vi "AlliGator Global Decay Fit Output String.vi"(0 "Plot Names":string[](array[string]), 5 "Fit Output":T2={"best nonlinear fit"=[], "best fit parameters"=[], "R^2"=0.0, "RMSE"=0.0, "error out"={"status"=FALSE, "code"=0, "source"=""}, "Fitting Method"=enum."Least Square", "number of function calls"=0, "number of iterations"=0, "covariance"=[], "Chi 2"=0.0, "DOF"=0, "Fit Convergence Criterion"=enum."Continue", "Fitting Algorithm"=enum."Levenberg-Marquardt", "Weighted Fit"=enum."Unweighted", "Gradient"=0.0, "|Delta Chi 2|"=0.0, "|Delta Chi 2|/Chi 2"=0.0, "Max |Delta a| /|a|"=0.0, "Lambda"=-1.0, "RSS"=0.0, "AIC"=0.0, "BIC"=0.0, "Max number of function calls"=0, "Max number of iterations"=0, "IRF"={"X Array"=[], "Y Array"=[]}, "IRF Normalization Factor"=0.0, "Decay Normalization Factor"=0.0, "Number of offset fits"=0, "Weighted Chi2"=-1.0, "Unweighted Chi2"=-1.0}, 7 "Delta Best Fit Parameters":dbl[](array[numeric]), 9 "elapsed (relative) seconds":dbl, 11 "Error In":errorcluster, 12 "Fit Options":T9={"Show Fit Residuals"=TRUE, "Fit Model"=enum."1-Exponential", "Residual Type"=enum."Standard", "Max Decay Percentile"=0.0, "Min Decay Percentile"=0.0, "Show Full Decay"=TRUE, "Weights"=enum."Unweighted", "Fitting Method"=enum."Least Square", "Compute Parameter Uncertainties"=TRUE, "Periodic Boundaries"=TRUE, "Model Calculation"=enum."Simulation", "Period"=1.2500000000000001e-08, "Termination Criteria"={"Max Iterations"=1000, "Max Function Calls"=0, "Max Time"=1000.0, "Function Tolerance"=1e-06, "Parameter Tolerance"=1e-06, "Gradient Tolerance"=0.0, "Min Lambda"=1e-06, "Max Lambda"=1e-06, "Initial Tick Count"=0}, "Offset Resolution"=1.2500000000000001e-08, "Use Local IRF"=TRUE, "Fitting Algorithm"=enum."Levenberg-Marquardt", "Show Confidence Interval "=TRUE, "Confidence Level"=95.0} {"Confidence Level" min=0.0 max=100.0; "Offset Resolution" min=0.0; "Period" min=0.0; "Min Decay Percentile" min=0.0 max=1.0; "Max Decay Percentile" min=0.0 max=100.0}, 13 "Fit Parameter Constraints":T14[](array[typedef]) {"Max Value" format="%#.3g"; "Min Value" format="%#.3g"}, 14 "Global Fit Parameter Info":T8) -> (4 "Fit Output Message":string, 15 "Error Out":errorcluster)   [LabVIEW 2021, in "AlliGator Global Decay Fit.lvlib"]
uses:
  AlliGator Global Decay Fit.lvlib
  Decay Fit/AlliGator Decay Fit Parameter Constraints 2.ctl
  Fits/IRF(X)PSED/Decay Fit Parameters In List.ctl
  Fits/Decay Convolution/Decay Model.ctl
  Fits/Residual Type.ctl
  Fits/Non-linear Fitting Method v2.ctl
  Fits/Fit Calculation Method.ctl
  Fits/Non-linear Fitting Algorithm.ctl
  Fits/Global Fits/Global Fit Parameters Information.ctl
  Fits/Non-linear Fit Output v4.ctl
  Fits/Nonlinear Fit Method.ctl
  <vilib>/Analysis/Matrix/Datatypes/RealMatrix.ctl
  Fits/Convergence Criteria.ctl
  Fits/IRF(X)PSED/Fit Weights Type v2.ctl
  Graphs/XY Graph/XY Graph Plot Data.ctl
  Settings/AlliGator Settings List.ctl
  <vilib>/Utility/error.llb/DialogType.ctl
  dade2e8c-81fa-42a5-b12d-40fd9ae52111.vi
  Variant/Variant to Data/Variant to Boolean.vi
  <vilib>/Utility/libraryn.llb/Get File Extension.vi
  <vilib>/Utility/error.llb/Error Cluster From Error Code.vi
  <vilib>/ErrorRing/Error Ring.xnode
  Fits/Fits.lvlib
  Strings/Strings.lvlib
  Settings/AlliGator Settings.lvlib
  Variant/Variant to Data/Variant to Data.lvlib
  Sound/Sound.lvlib
  Decay Fit/AlliGator Decay Fit.lvlib
  <vilib>/Analysis/Matrix/NI_Matrix.lvlib
  Graphs/XY Graph/XY Graph Add-Ons.lvlib
  Fits/IRF(X)PSED/Decay Fit Options v4.ctl
panel:
  in  "NL Fit Method":T1
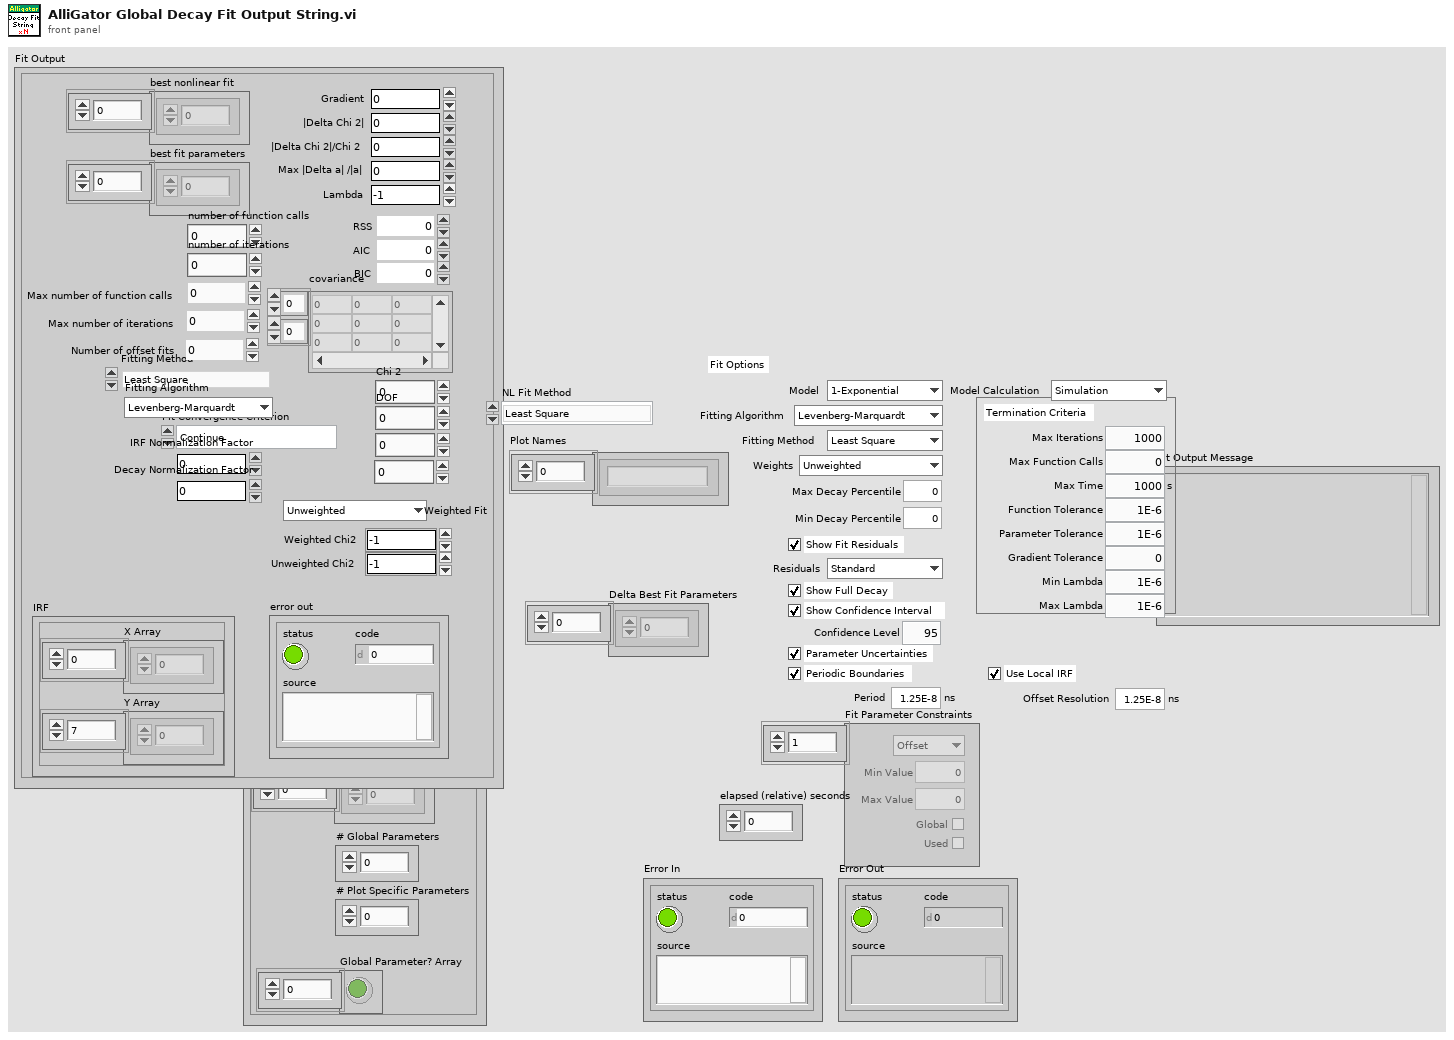
[diagram p1: front panel]
types:
  T1 = typedef "Fits.lvlib/Nonlinear Fit Method.ctl" = enum16{"Least Square", "Least Absolute Residual", "Bisquare", "MLE"}
  T2 = typedef "Fits.lvlib/Non-linear Fit Output v4.ctl" = cluster{"best nonlinear fit":dbl[], "best fit parameters":dbl[], "R^2":dbl, "RMSE":dbl, "error out":errorcluster, "Fitting Method":T1, "number of function calls":i32, "number of iterations":i32, "covariance":T3, "Chi 2":dbl, "DOF":i32, "Fit Convergence Criterion":T4, "Fitting Algorithm":T5, "Weighted Fit":T6, "Gradient":dbl, "|Delta Chi 2|":dbl, "|Delta Chi 2|/Chi 2":dbl, "Max |Delta a| /|a|":dbl, "Lambda":dbl, "RSS":dbl, "AIC":dbl, "BIC":dbl, "Max number of function calls":i32, "Max number of iterations":i32, "IRF":T7, "IRF Normalization Factor":dbl, "Decay Normalization Factor":dbl, "Number of offset fits":i32, "Weighted Chi2":dbl, "Unweighted Chi2":dbl}
  T3 = typedef "NI_Matrix.lvlib/RealMatrix.ctl" = dbl[][]
  T4 = typedef "Fits.lvlib/Convergence Criteria.ctl" = enum16{"Continue", "Tolerances Exceeded", "Max Time Exceeded", "Max Iterations Exceeded", "Max Function Evaluations Exceeded", "Scale Range Exceeded"}
  T5 = typedef "Fits.lvlib/Non-linear Fitting Algorithm.ctl" = enum16{"Levenberg-Marquardt", "Trust-Region Dogleg"}
  T6 = typedef "Fits.lvlib/Fit Weights Type v2.ctl" = enum16{"Unweighted", "1/Variance (Neyman)", "1/Variance (Pearson)", "Best of All"}
  T7 = typedef "XY Graph Add-Ons.lvlib/XY Graph Plot Data.ctl" = cluster{"X Array":dbl[], "Y Array":dbl[]}
  T8 = typedef "Fits.lvlib/Global Fit Parameters Information.ctl" = cluster{"Original Parameter Indices":i32[], "# Global Parameters":i32, "# Plot Specific Parameters":i32, "Global Parameter? Array":bool[]}
  T9 = typedef "Fits.lvlib/Decay Fit Options v4.ctl" = cluster{"Show Fit Residuals":bool, "Fit Model":T10, "Residual Type":T11, "Max Decay Percentile":dbl, "Min Decay Percentile":dbl, "Show Full Decay":bool, "Weights":T6, "Fitting Method":T12, "Compute Parameter Uncertainties":bool, "Periodic Boundaries":bool, "Model Calculation":T13, "Period":dbl[unit], "Termination Criteria":cluster{"Max Iterations":i32, "Max Function Calls":i32, "Max Time":dbl[unit], "Function Tolerance":dbl, "Parameter Tolerance":dbl, "Gradient Tolerance":dbl, "Min Lambda":dbl, "Max Lambda":dbl, "Initial Tick Count":u32}, "Offset Resolution":dbl[unit], "Use Local IRF":bool, "Fitting Algorithm":T5, "Show Confidence Interval ":bool, "Confidence Level":dbl}
  T10 = typedef "Fits.lvlib/Decay Model.ctl" = enum16{"1-Exponential", "2-Exponentials"}
  T11 = typedef "Fits.lvlib/Residual Type.ctl" = enum16{"Standard", "Normalized", "Reduced"}
  T12 = typedef "Fits.lvlib/Non-linear Fitting Method v2.ctl" = enum16{"Least Square", "Least Absolute Residual", "Bisquare", "MLE", "-", "Best of All"}
  T13 = typedef "Fits.lvlib/Fit Calculation Method.ctl" = enum16{"Simulation", "Convolution", "Integration"}
  T14 = typedef "AlliGator Decay Fit.lvlib/AlliGator Decay Fit Parameter Constraints 2.ctl" = cluster{"Fit Parameter":T15, "Min Value":dbl, "Max Value":dbl, "Global":bool, "Used":bool}
  T15 = typedef "Fits.lvlib/Decay Fit Parameters In List.ctl" = enum16{"Offset", "Baseline", "A_1", "tau_1", "A_2", "tau_2"}
  T16 = typedef "AlliGator Settings.lvlib/AlliGator Settings List.ctl" = enum16{"GUI:Visible Settings Tab", "GUI:Last Run Version", "Source Image:Use Image Histogram for Contrast", "Source Image:Low Count Pixels Rejection Options", "Source Image:High Count Pixels Rejection Options", "Source Image:Use Image Brightness", "Source Image:Blend Overlay with Image Background", "Source Image:Use Fixed ROI Diameter", "Source Image:ROI Diameter", "Source Image:ROI Center Color", "Source Image:Peak Threshold", "Source Image:Intensity Threshold", "Source Image:Image Binning Options", "Source Image:Image Smoothing Options", "Source Image:Image Histogram Active", "Source Image:Invert Binary Mask", "Source Image:Hot Pixel Removal", "Source Image:Overlay Analyzed ROI Center", "Source Image:Auto-Adjust Contrast", "Source Image:Histogram Lower Percentile", "Source Image:Histogram Upper Percentile", "Source Image:Save Source Image", "Source Image:Scale Bar Options", "Source Image:Image Resolution (Pixel Size)", "Source Image:Flatfield Correction", "Source Image:Show Dead Left Columns Correction", "Source Image:Dead Left Columns Correction", "Source Image:Image Pre-Processing Operations Order", "Source Image:Overlay ROI Median", "Source Image:Median Overlay Color", "Data Information:Gate Width", "Data Information:Nanotime Gate Separation", "Data Information:Macrotime Gate Separation", "Data Information:Gate Step", "Data Information:# Gates", "Data Information:Gate Image Exposure", "Data Information:Gate Image Integration", "Data Information:Gates to Skip", "Data Information:Gates to Keep", "Data Information:Define Gates to", "Data Information:Channel Name", "Data Information:Available Channel Names", "Data Information:Channel Arithmetic", "Data Information:Background File Subtraction", "Data Information:Background File", "Data Information:Background Scaling Factor", "Data Information:Background Pile-up Correction", "Data Information:Background Pixel Well Capacity", "Data Information:Laser Period", "Data Information:SYNC Period", "Data Information:Pile-up Correction", "Data Information:Pixel Well Capacity", "Data Information:Dataset Scaling Factor", "Fluorescence Decay_Decay Pre-Processing:Reverse Gates", "Fluorescence Decay_Decay Pre-Processing:Verbose Decay Pre-Processing", "Fluorescence Decay_Decay Pre-Processing:Use Decay Pre-Processing", "Fluorescence Decay_Decay Pre-Processing:Background Subtraction", "Fluorescence Decay_Decay Pre-Processing:Background Definition Range", "Fluorescence Decay_Decay Pre-Processing:Baseline Subtraction Method", "Fluorescence Decay_Decay Pre-Processing:Decay Pre-Processing Operations Order", "Fluorescence Decay_Decay Pre-Processing:Smoothing Parameter", "Fluorescence Decay_Decay Pre-Processing:Shift Decay", "Fluorescence Decay_Decay Pre-Processing:Decay Shift Parameters", "Fluorescence Decay_Decay Pre-Processing:Fold Decay", "Fluorescence Decay_Decay Pre-Processing:# Folds", "Fluorescence Decay_Decay Pre-Processing:1-Normalize Decay", "Fluorescence Decay_Decay Pre-Processing:[0-1]-Normalize Decay", "Fluorescence Decay_Decay Pre-Processing:Smoothen Decay", "Fluorescence Decay_Decay Pre-Processing:Extrapolate Decay", "Fluorescence Decay_Decay Pre-Processing:Use Periodicity", "Fluorescence Decay_Decay Pre-Processing:Use Cursors", "Fluorescence Decay_Decay Pre-Processing:Tail Fraction", "Fluorescence Decay_Decay Pre-Processing:Head Fraction", "Fluorescence Decay_Decay Pre-Processing:Additional Points", "Fluorescence Decay_Decay Pre-Processing:Straighten Decay", "Fluorescence Decay_Decay Pre-Processing:Constant Background", "Fluorescence Decay_Decay Pre-Processing:Pixel-Normalize Decay", "Fluorescence Decay_Advanced Analysis:Extract IRF instead of Decay", "Fluorescence Decay_Advanced Analysis:IRF Extraction Options", "Fluorescence Decay_Advanced Analysis:IRF Optimization Options", "Fluorescence Decay_Advanced Analysis:Square Pulse Options", "Fluorescence Decay_Advanced Analysis:IRF Order", "Fluorescence Decay_Advanced Analysis:IRF Time Constants", "Fluorescence Decay_Advanced Analysis:Wavelet Analysis Options", "Fluorescence Decay_Advanced Analysis:Average Lifetime Options", "Fluorescence Decay_Fit Options:Fit Options", "Fluorescence Decay_Fit Options:Use Legacy Fitting Approach", "Fluorescence Decay_Fit Options:Use Data Information Laser Period", "Fluorescence Decay_Fit Parameters:Displayed Fit Parameters", "Fluorescence Decay_Fit Parameters:Fit Parameter Constraints", "Fluorescence Decay_Fit Parameters:Export Tabulated Results", "Fluorescence Decay_Fit Parameters:MLE Baseline Offset Type", "Fluorescence Decay_Fit Parameters:MLE Baseline Offset", "Fluorescence Decay_Fit Parameters:Guess Parameter Names", "Fluorescence Decay_Fit Parameters:Guess Parameter Values", "Fluorescence Decay_Fit Parameters:Guess Parameters Options", "Fluorescence Decay_Fit Parameters:Optimal Offset Selection Criterion", "Fluorescence Decay_Styles:Show Last Decay Only", "Fluorescence Decay_Styles:Decay Graph Color Array", "Fluorescence Decay:Decay Graph Active", "Fluorescence Decay Statistics:Min Peak Value", "Fluorescence Decay Statistics:Reject Low Decay Peak Pixels", "Fluorescence Decay Statistics:Reject High Decay Peak Pixels", "Fluorescence Decay Statistics:Max Peak Value", "Time Traces:Use File Timestamp", "Time Traces:Time Step", "Time Traces:Use Intensity Correction File", "Time Traces:Intensity Correction File", "Phasor Plot:Phasor Plot Smoothing Options", "Phasor Plot:Phasor Plot Size", "Phasor Plot:Phasor Plot Graphics Options", "Phasor Plot:Cumulative Phasor Plot", "Phasor Plot:Use Phasor Brightness", "Phasor Plot:Blend Overlay with Phasor Background", "Phasor Plot:Save Phasor Plot", "Phasor Plot:Show References", "Phasor Plot:Phasor Ratio Decay Range", "Phasor Plot:Exponential Fading", "Phasor Plot:Phasor Ratio Reference Colors", "Phasor Plot:Reference Radius", "Phasor Plot:Show Color Map Vertices", "Phasor Plot:Phasor Plot Active", "Phasor Plot:Phasor Ratio Color Map Type", "Phasor Plot:Phasor Ratio Color Map", "Phasor Plot:Phasor Ratio Display Range", "Phasor Plot:Selected Image ROI(s)", "Phasor Plot:All Image ROIs", "Phasor Plot:Selected Phasor Plot ROI(s)", "Phasor Plot:All Phasor Plot ROIs", "Phasor Plot:Phasor Ratio Color-Coded Quantity", "Phasor Plot:Store Phasor Harmonics", "Phasor Plot:Draw Reference Segment", "Phasor Plot:User-Defined Quantity", "Phasor Plot:Color Scale High Color", "Phasor Plot:Color Scale Low Color", "Phasor Plot:Intensity-weighted Phasor Plot", "Phasor Graph:Phasor Frequency", "Phasor Graph:Phasor Ratio Type", "Phasor Graph:Pixel-level Phasor Computation", "Phasor Graph:Save Phasor Graph", "Phasor Graph:Phasor Graph Active", "Phasor Graph:Phasor SDV Options", "Phasor Graph:Intensity-weighted Phasor Graph", "Phasor Graph:Define Shortest Lifetime as", "Phasor Calibration:Use Backup Calibration if needed", "Phasor Calibration:Backup Calibration Type", "Phasor Calibration:Calibration Type", "Phasor Calibration:Calibration Lifetime", "Phasor Calibration:Calibration Map Algorithm", "Single-Exponential Phasor Locus (SEPL):Gate Parameters", "Single-Exponential Phasor Locus (SEPL):User-defined Gate", "Single-Exponential Phasor Locus (SEPL):User-defined IRF", "Single-Exponential Phasor Locus (SEPL):Phasor Parameters", "Single-Exponential Phasor Locus (SEPL):Decay & IRF Parameters", "Single-Exponential Phasor Locus (SEPL):Display Parameters", "Lifetime Analysis:Decay Analysis Parameters", "Lifetime Analysis:Lifetime Map Active", "Plugins:Python Settings", "Miscellaneous:Verbose Mode", "Miscellaneous:Beep after Script", "Miscellaneous:Saved Image File Format", "Miscellaneous:Exported Gate Image Settings", "Miscellaneous:Include Loading in Timing", "Miscellaneous:Verbose Settings Mode", "Miscellaneous:Histogram Options", "Miscellaneous:Beep on Error", "Miscellaneous:# Logical Processors Used", "Miscellaneous:ROI Description Max Characters", "Miscellaneous:Verbose Error Mode", "Miscellaneous:Transparent Mask Color"}
  T17 = typedef "DialogType.ctl" = u16
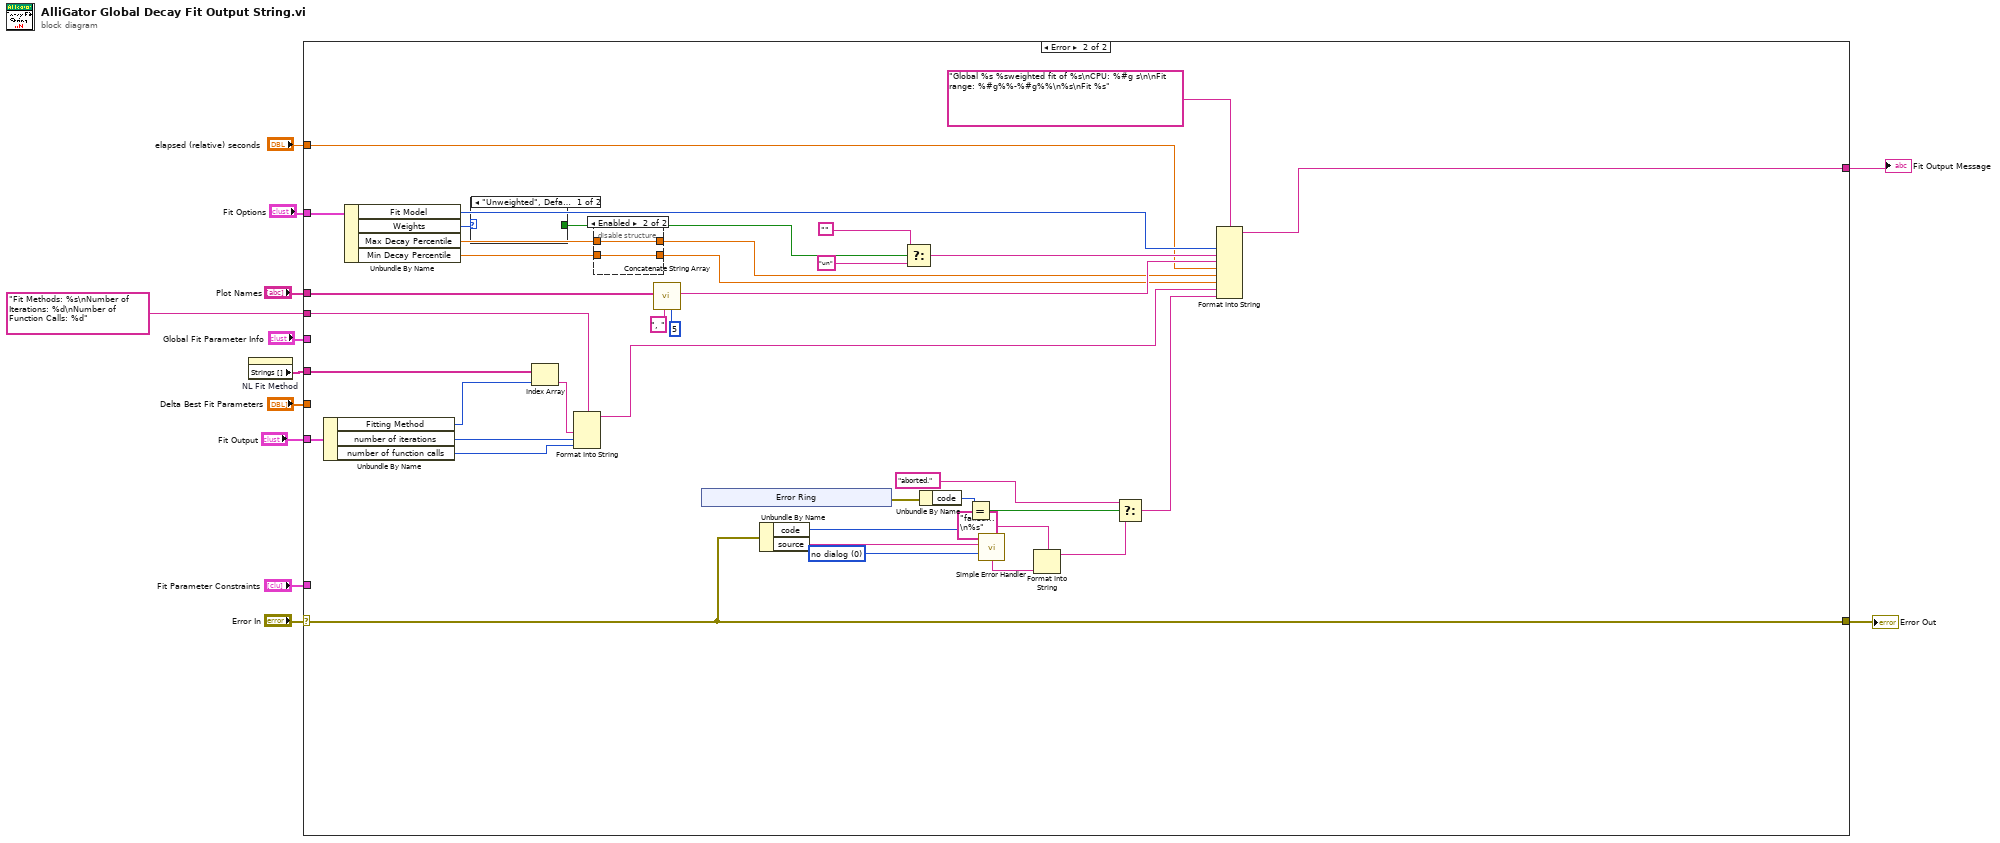
[diagram p0: block diagram]
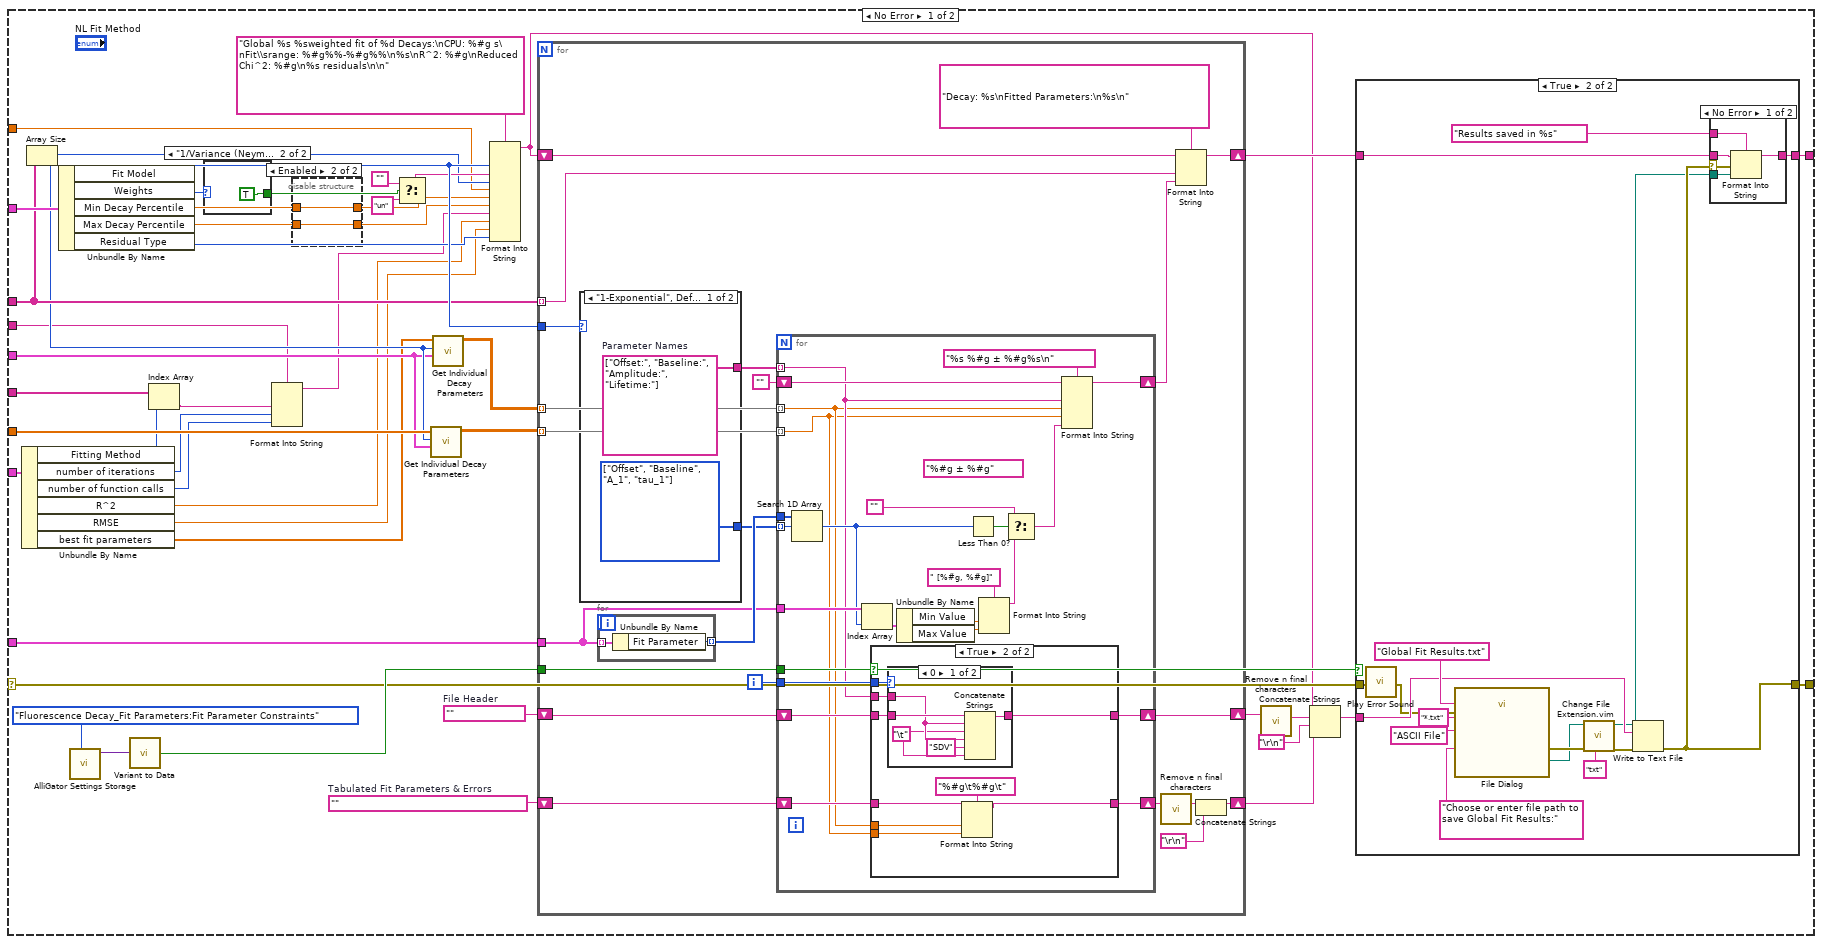
[diagram p2: hidden frame]
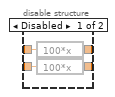
[diagram p3: hidden frame]
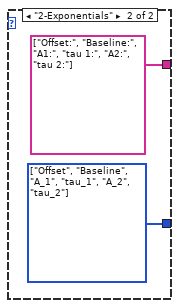
[diagram p7: hidden frame]
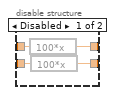
[diagram p10: hidden frame]
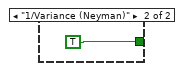
[diagram p11: hidden frame]
diagram:
  n1 = property on="NL Fit Method" class="Enum (strict)"() -> ("Strings []"=w2:string[])  [unwired: 2 in, 2 out]
  n2 = case shown="Error" "Error In" {
    selector: "Error In" -> [w31 w187]
    tunnel: "Plot Names" -> [w47 w190]
    tunnel: "Delta Best Fit Parameters" -> [w45 _]
    tunnel: "Fit Options" -> [w57 w197]
    tunnel: [w28 w196] -> w10
    tunnel: "Fit Parameter Constraints" -> [w59 _]
    tunnel: "Global Fit Parameter Info" -> [w43 _]
    tunnel: "elapsed (relative) seconds" -> [w41 w163]
    tunnel: [w30 w187] -> w4
    tunnel: "Fit Output" -> [w25 w164]
    tunnel: w2 -> [w16 w172]
    tunnel: "Fit Methods: %s\nNumber of Iterations: %d\nNumber of Function Calls: %d" ("format string") -> [w15 w171]
    frame No Error {
      w37 = ""  # File Header
      w38 = ""  # Tabulated Fit Parameters & Errors
      n3 = Unbundle By Name(w25) -> ("Fitting Method"=w21:T1, "number of iterations"=w19:i32, "number of function calls"=w18:i32, "R^2"=w23:dbl, "RMSE"=w22:dbl, "best fit parameters"=w24:dbl[])
      n4 = Array Size(array=w47) -> (size(s)=w44:i32)
      n5 = Unbundle By Name(w57) -> ("Fit Model"=w54:T10, "Weights"=w14:T6, "Min Decay Percentile"=w56:dbl, "Max Decay Percentile"=w55:dbl, "Residual Type"=w48:T11)
      n6 = call "AlliGator Settings Storage.vi"("AlliGator Settings List"=AlliGator_Settings_List."Fluorescence Decay_Fit Parameters:Fit Parameter Constraints") -> ("Variant Data out"=w39:variant)  [unwired: 9 in, 1 out]
      n7 = call-poly "Variant to Data.vi"("Variant"=w39) -> ("Value"=w33:bool)  [unwired: 8 in]
      n8 = Index Array(array=w16, index=w21) -> (element=w20:string)
      n9 = case shown="\"1/Variance (Neyman)\"" w14 {
        tunnel: [_ TRUE ("Weighted Fit")] -> w13
        frame "Unweighted", Default {
        }
        frame "1/Variance (Neyman)" {
        }
      }
      n10 = Format Into String(format string=w15, w20, w19, w18) -> (resulting string=w17:string)  [unwired: 2 in, 1 out]
      n11 = disable-structure shown="Enabled" {
        disable-tunnel: w56 -> [w63 w65]
        disable-tunnel: w55 -> [w62 w64]
        disable-tunnel: [w61 w65] -> w50
        disable-tunnel: [w60 w64] -> w49
        frame Disabled {
          n12 = expression code="100*x"(w63) -> (w61:dbl)
          n13 = expression code="100*x"(w62) -> (w60:dbl)
        }
        frame Enabled {
        }
      }
      n14 = Select(t="", s=w13, f="un") -> (s? t:f=w51:string)
      n15 = call "Get Individual Decay Parameters.vi"("Global Fit Parameter Info"=w43, "# Decays"=w44, "Global Fit Parameters Array"=w45) -> ("All Parameters Array"=w42:dbl[][])  [unwired: 5 in, 3 out]
      n16 = call "Get Individual Decay Parameters.vi"("Global Fit Parameter Info"=w43, "# Decays"=w44, "Global Fit Parameters Array"=w24) -> ("All Parameters Array"=w46:dbl[][])  [unwired: 5 in, 3 out]
      n17 = Format Into String(format string="Global %s %sweighted fit of %d Decays:\nCPU: %#g s\nFit\\srange: %#g%%-%#g%%\n%s\nR^2: %#g\nReduced Chi^2: %#g\n%s residuals\n\n", w54, w51, w44, w41, w50, w49, w17, w23, w22, w48) -> (resulting string=w27:string)  [unwired: 2 in, 1 out]
      n18 = for {
        tunnel: w47 -> [w101] mode=indexing
        tunnel: w42 -> [w111] mode=indexing
        tunnel: w59 -> [w105]
        shift-right: [w109] -> w29
        shift-left: w27 -> [w104]
        tunnel: w54 -> [w103]
        tunnel: w46 -> [w100] mode=indexing
        tunnel: w33 -> [w98]
        shift-right: [w92] -> w34
        shift-left: w38 -> [w97]
        shift-right: [w95] -> w36
        shift-left: w37 -> [w96]
        i -> [w99]
        n19 = case shown="\"1-Exponential\", Default" w103 {
          tunnel: [w116 string[] ["Offset:", "Baseline:", "A1:", "tau 1:", "A2:", "tau 2:"] ("Parameter Names")] -> w110
          tunnel: [w115 w117] -> w106
          frame "1-Exponential", Default {
            w115 = T15[] [enum."Offset", enum."Baseline", enum."A_1", enum."tau_1"] items=["Offset", "Baseline", "A_1", "tau_1", "A_2", "tau_2"] ("Array")
            w116 = string[] ["Offset:", "Baseline:", "Amplitude:", "Lifetime:"]  # Parameter Names
          }
          frame "2-Exponentials" {
            w117 = T15[] [enum."Offset", enum."Baseline", enum."A_1", enum."tau_1", enum."A_2", enum."tau_2"] items=["Offset", "Baseline", "A_1", "tau_1", "A_2", "tau_2"] ("Array")
          }
        }
        n20 = for {
          tunnel: w105 -> [w114] mode=indexing
          tunnel: [w113] -> w107 mode=indexing
          n21 = Unbundle By Name(w114) -> ("Fit Parameter"=w113:T15)
        }
        n22 = for {
          tunnel: w100 -> [w120] mode=indexing
          tunnel: w111 -> [w119] mode=indexing
          tunnel: w110 -> [w124] mode=indexing
          shift-right: [w142] -> w102
          shift-left: "" -> [w141]
          tunnel: w107 -> [w139]
          tunnel: w106 -> [w138] mode=indexing
          tunnel: w105 -> [w137]
          tunnel: w99 -> [w125]
          tunnel: w98 -> [w127]
          shift-right: [w121] -> w93
          shift-left: w97 -> [w126]
          shift-right: [w122] -> w95
          shift-left: w96 -> [w123]
          (unwired) "%#g ± %#g" ("format string")
          n23 = Search 1D Array(1D array=w139, element=w138) -> (index of element=w128:i32)  [unwired: 1 in]
          n24 = Index Array(array=w137, index=w128) -> (element=w132:T14)
          n25 = case shown="True" w127 {
            tunnel: w126 -> [w143 w149]
            tunnel: w125 -> [_ w153]
            tunnel: w124 -> [_ w152]
            tunnel: w123 -> [w144 w151]
            tunnel: [w144 w150] -> w122
            tunnel: [w143 w148] -> w121
            tunnel: w120 -> [_ w146]
            tunnel: w119 -> [_ w145]
            frame False {
            }
            frame True {
              n26 = case shown="0" w153 {
                tunnel: w152 -> [w156 _]
                tunnel: w151 -> [w158 w159]
                tunnel: [w157 w159] -> w150
                frame 0 {
                  w154 = "\t"
                  n27 = Concatenate Strings(w158, w156, w154, w156, "SDV" ("string"), w154) -> (w157:string)
                }
                frame 1, Default {
                }
              }
              n28 = Format Into String(format string="%#g\t%#g\t", initial string=w149, w146, w145) -> (resulting string=w148:string)  [unwired: 1 in, 1 out]
            }
          }
          n29 = Unbundle By Name(w132) -> ("Min Value"=w131:dbl, "Max Value"=w130:dbl)
          n30 = Less Than 0?(x=w128) -> (x < 0?=w136:bool)
          n31 = Format Into String(format string=" [%#g, %#g]", w131, w130) -> (resulting string=w129:string)  [unwired: 2 in, 1 out]
          n32 = Select(t="", s=w136, f=w129) -> (s? t:f=w134:string)
          n33 = Format Into String(format string="%s %#g ± %#g%s\n", initial string=w141, w124, w120, w119, w134) -> (resulting string=w142:string)  [unwired: 1 in, 1 out]
        }
        n34 = call "Remove n final characters.vi"("String in"=w93) -> ("String out"=w94:string)  [unwired: 8 in]
        n35 = Format Into String(format string="Decay: %s\nFitted Parameters:\n%s\n", initial string=w104, w101, w102) -> (resulting string=w109:string)  [unwired: 1 in, 1 out]
        n36 = Concatenate Strings(w94, "\r\n") -> (w92:string)
      }
      n37 = call "Remove n final characters.vi"("String in"=w36) -> ("String out"=w35:string)  [unwired: 8 in]
      n38 = Concatenate Strings(w27, w35, "\r\n", w34) -> (w32:string)
      n39 = case shown="True" w33 {
        tunnel: w32 -> [_ w76]
        tunnel: w31 -> [w68 w70]
        tunnel: [w68 w77] -> w30
        tunnel: w29 -> [w67 w84]
        tunnel: [w67 w83] -> w28
        frame False {
        }
        frame True {
          n40 = call "Play Error Sound.vi"("Error In"=w70) -> ("Error Out"=w71:errorcluster)  [unwired: 26 in]
          n41 = call "File Dialog"("prompt"="Choose or enter file path to save Global Fit Results:" ("prompt (Choose or enter file path)"), "default name"="Global Fit Results.txt", "error in"=w71, "pattern (all files)"="*.txt", "pattern label"="ASCII File") -> ("selected path"=w69:path, "error out"=w75:errorcluster)  [unwired: 7 in, 2 out]
          n42 = call "Change File Extension.vim"("File Extension"="txt", "error in (no error)"=w75, "File in"=w69) -> ("error out"=w74:errorcluster, "File out"=w72:path)  [unwired: 7 in]
          n43 = Write to Text File(file (use dialog)=w72, text=w76, error in=w74) -> (error out=w77:errorcluster)  [unwired: 1 in, 2 out]
          n44 = case shown="No Error" w77 {
            selector: w77 -> [w87 _]
            tunnel: w84 -> [w89 w90]
            tunnel: w72 -> [w88 _]
            tunnel: [w86 w90] -> w83
            tunnel: "Results saved in %s" ("format string") -> [w85 _]
            frame No Error {
              n45 = Format Into String(format string=w85, initial string=w89, error in=w87, w88) -> (resulting string=w86:string)  [unwired: 1 out]
            }
            frame Error {
            }
          }
        }
      }
    }
    frame Error {
      w179 = T17 0 items=["no dialog", "OK message", "continue or stop message", "OK message + warnings", "continue/stop + warnings"] ("type of dialog (OK msg:1)")
      n46 = Unbundle By Name(w164) -> ("Fitting Method"=w173:T1, "number of iterations"=w175:i32, "number of function calls"=w176:i32)
      n47 = Unbundle By Name(w197) -> ("Fit Model"=w194:T10, "Weights"=w161:T6, "Max Decay Percentile"=w178:dbl, "Min Decay Percentile"=w177:dbl)
      n48 = case shown="\"Unweighted\", Default" w161 {
        tunnel: [_ TRUE ("Weighted Fit")] -> w160
        frame "Unweighted", Default {
        }
        frame "1/Variance (Neyman)" {
        }
      }
      n49 = Index Array(array=w172, index=w173) -> (element=w174:string)
      n50 = Format Into String(format string=w171, w174, w175, w176) -> (resulting string=w168:string)  [unwired: 2 in, 1 out]
      n51 = disable-structure shown="Enabled" {
        disable-tunnel: w178 -> [w201 w203]
        disable-tunnel: w177 -> [w200 w202]
        disable-tunnel: [w199 w203] -> w170
        disable-tunnel: [w198 w202] -> w169
        frame Disabled {
          n52 = expression code="100*x"(w201) -> (w199:dbl)
          n53 = expression code="100*x"(w200) -> (w198:dbl)
        }
        frame Enabled {
        }
      }
      n54 = call "Concatenate String Array.vi"("Max Number of Elements (None: -1)"=5 ("Max Number of Elements (None: 1)"), "Separator (TAB)"=", ", "String Array"=w190) -> ("Formatted String"=w188:string)  [unwired: 8 in]
      n55 = xnode "Error Ring"() -> ("error out"=w186:errorcluster)
      n56 = Unbundle By Name(w187) -> ("code"=w180:i32, "source"=w181:string)
      n57 = Select(t="", s=w160, f="un") -> (s? t:f=w191:string)
      n58 = Unbundle By Name(w186) -> ("code"=w185:i32)
      n59 = Equal?(x=w185, y=w180) -> (x = y?=w184:bool)
      n60 = call <vilib>:"Simple Error Handler.vi"("error code (no error:0)"=w180, "error source (\" \")"=w181, "type of dialog (OK msg:1)"=w179) -> ("message"=w166:string)  [unwired: 2 in, 4 out]
      n61 = Format Into String(format string="failed...\n%s", w166) -> (resulting string=w165:string)  [unwired: 2 in, 1 out]
      n62 = Select(t="aborted.", s=w184, f=w165) -> (s? t:f=w182:string)
      n63 = Format Into String(format string="Global %s %sweighted fit of %s\nCPU: %#g s\n\nFit range: %#g%%-%#g%%\n%s\nFit %s", w194, w191, w188, w163, w170, w169, w168, w182) -> (resulting string=w196:string)  [unwired: 2 in, 1 out]
    }
  }
  "Fit Output Message" <- w10
  "Error Out" <- w4
